vi "FullAlign.vi"(0 "Joystick 0":dbl, 1 "Button":bool=TRUE, 5 "Joystick 1":dbl, 7 "Distance":dbl=23.73829999999998, 9 "Angle":dbl=57.28800997198897) -> (4 "Right Motor":dbl, 6 "Left Motor":dbl=-0.0, 15 "In Range?":bool)   [LabVIEW 2016]
panel:
  out "Sees Target?":bool=TRUE
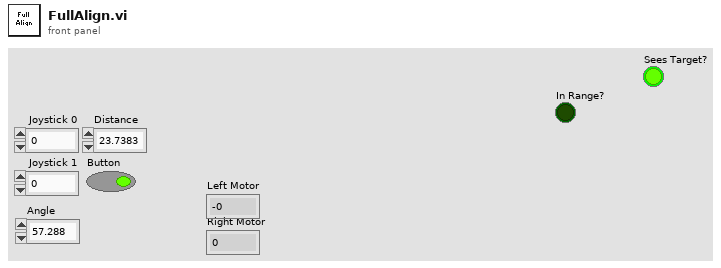
[diagram p1: front panel]
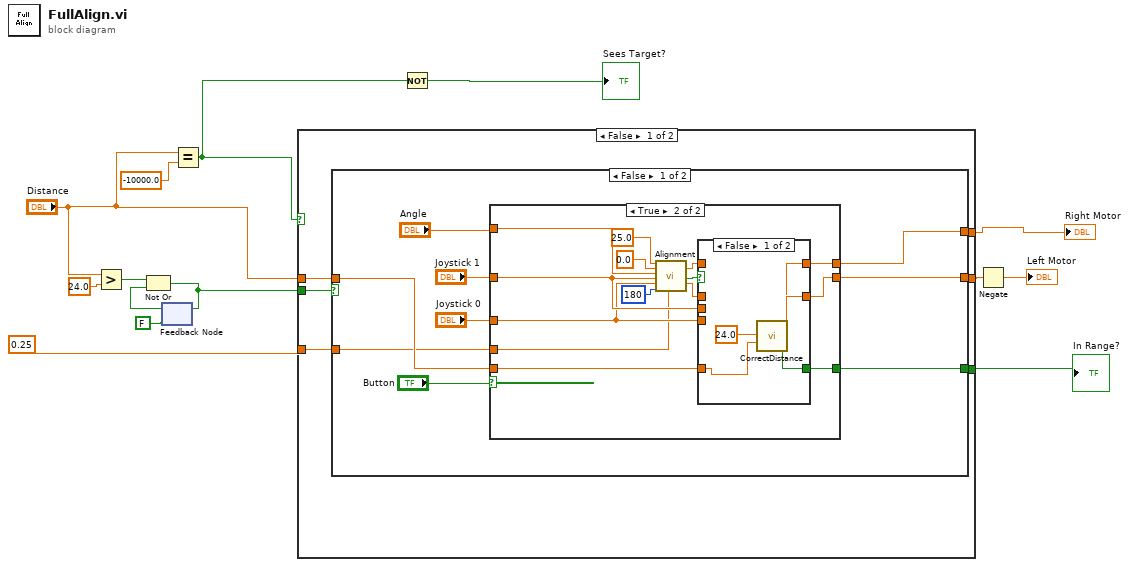
[diagram p0: block diagram]
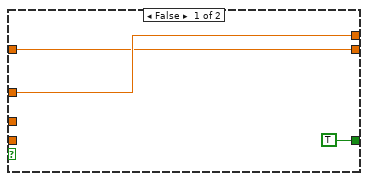
[diagram p2: hidden frame]
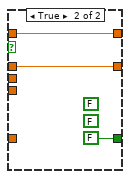
[diagram p3: hidden frame]
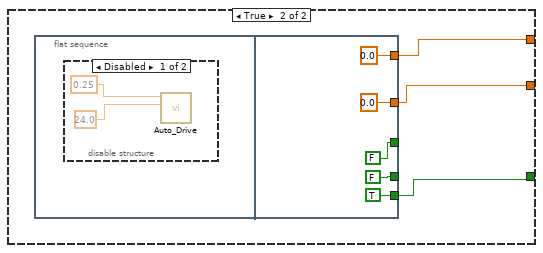
[diagram p4: hidden frame]
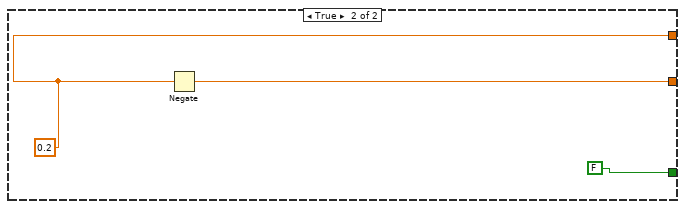
[diagram p6: hidden frame]
diagram:
  n1 = Greater?(x="Distance", y=24.0) -> (0:w11:bool)
  n2 = feedback #1(FALSE) -> (w12:bool)
  n3 = Not Or(1:w12, 2:w11) -> (0:w10:bool)
  n4 = feedback-in #1(w10) -> ()
  n5 = Equal?(x="Distance", y=-10000.0) -> (x = y?=w7:bool)
  n6 = case shown="False" w7 {
    tunnel: w10 -> [w20 _]
    tunnel: [w19 w65] -> w2
    tunnel: [w18 w66] -> w3
    tunnel: [w17 FALSE] -> w9
    tunnel: "Distance" -> [w16 _]
    tunnel: 0.25 -> [w15 _]
    frame False {
      n7 = case shown="False" w20 {
        tunnel: w16 -> [w25 _]
        tunnel: [w24 w56] -> w19
        tunnel: [w23 w55] -> w18
        tunnel: [w22 w57] -> w17
        tunnel: w15 -> [w21 _]
        frame False {
          n8 = case shown="True" "Button" {
            tunnel: "Joystick 1" -> [w31 w41]
            tunnel: "Joystick 0" -> [w32 w40]
            tunnel: [w31 w46] -> w23
            tunnel: [w32 w45] -> w24
            tunnel: "Angle" -> [_ w43]
            tunnel: [TRUE w36] -> w22
            tunnel: w25 -> [_ w35]
            tunnel: w21 -> [_ w33]
            frame False {
            }
            frame True {
              n9 = call "Alignment.vi"("Range"=25.0, "Target"=0.0, "Camera Feedback"=w43, "RightMotorSpeed"=w41, "LeftMotorSpeed"=w40, "POV"=180, "Turn_Gain"=w33) -> ("Right Motor"=w39:dbl, "LeftAndRight?"=w37:bool, "Left Motor"=w38:dbl)  [unwired: 10 in]
              n10 = case shown="False" w37 {
                tunnel: w41 -> [_ _]
                tunnel: w40 -> [_ _]
                tunnel: [w50 w53] -> w46
                tunnel: [w49 w54] -> w45
                tunnel: w39 -> [_ w54]
                tunnel: w38 -> [_ w53]
                tunnel: [w47 FALSE] -> w36
                tunnel: w35 -> [w48 _]
                frame False {
                  n11 = call "CorrectDistance.vi"("CenterPoint"=24.0, "Distance"=w48) -> ("In Range?"=w47:bool, "Right Motor"=w49:dbl, "Left Motor"=w50:dbl)  [unwired: 23 in]
                }
                frame True {
                  (unwired) FALSE
                  (unwired) FALSE
                }
              }
            }
          }
        }
        frame True {
          n12 = flat-sequence {
            tunnel: [FALSE] -> _
            tunnel: [FALSE] -> _
            tunnel: [TRUE] -> w57
            tunnel: [0.0] -> w56
            tunnel: [0.0] -> w55
            frame #0 {
              n13 = disable-structure shown="Disabled" {
                frame Disabled {
                  n14 = call "Auto_Drive.vi"("distance"=24.0, "Drive Effort"=0.25) -> ()  [unwired: 10 in]
                }
                frame Enabled {
                }
              }
            }
            frame #1 {
            }
          }
        }
      }
    }
    frame True {
      w65 = 0.2
      n15 = Negate(x=w65) -> (-x=w66:dbl)
    }
  }
  "Right Motor" <- w2
  "In Range?" <- w9
  n16 = Not(x=w7) -> (.not. x?=→"Sees Target?":bool)
  n17 = Negate(x=w3) -> (-x=→"Left Motor":dbl)
